vi "MicrowaveAmp.vi"(8 "error in (no error)":errorcluster, 11 "MicrowaveAmp in":refnum<class "MicrowaveAmp.lvclass">) -> (0 "error out":errorcluster, 3 "MicrowaveAmp out":refnum<class "MicrowaveAmp.lvclass">)   [LabVIEW 2009, in "MicrowaveAmp.lvclass"]
uses:
  MicrowaveAmp.lvclass
  Global/GPIB Numbers.vi
panel:
  out "Status":string
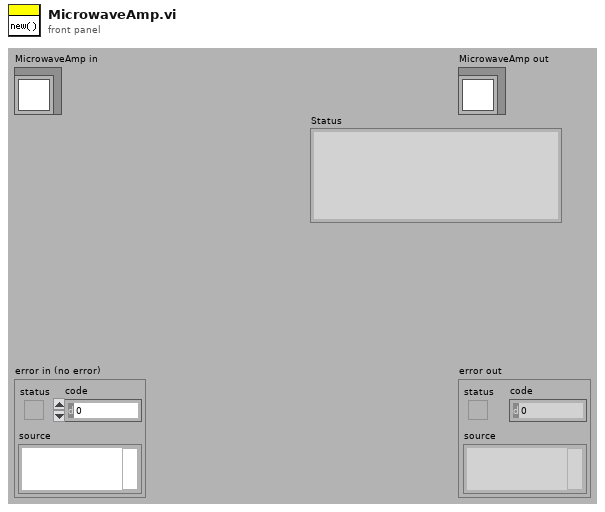
[diagram p1: front panel]
types:
  T1 = typedef "GPIB Type Def.ctl" = cluster{"Name":string, "bus":dbl, "GPIB":dbl, "GPIB as string":string, "byte":i32, "VISA Resource Name":refnum<visa-resource-name>}
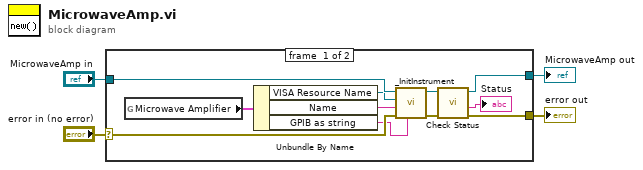
[diagram p0: block diagram]
diagram:
  n1 = case shown="No Error" "error in (no error)" {
    selector: "error in (no error)" -> [w13 w17]
    tunnel: [w11 w17] -> w3
    tunnel: [w9 w16] -> w1
    tunnel: "MicrowaveAmp in" -> [w14 w16]
    frame #0 {
      n2 = global read "GPIB Numbers.vi" "Microwave Amplifier"() -> (w15:T1)
      n3 = Unbundle By Name(w15) -> ("VISA Resource Name"=w7:refnum<visa-resource-name>, "Name"=w6:string, "GPIB as string"=w5:string)
      n4 = call-dynamic "_InitInstrument.vi"("GPIB as string"=w5, "error in (no error)"=w13, "Name"=w6, "VISA Resource Name"=w7, "Instrument in"=w14) -> ("error out"=w12:errorcluster, "Instrument out"=w10:refnum<class "MicrowaveAmp.lvclass">)  [unwired: 1 in, 4 out]
      n5 = call-dynamic "Check Status.vi"("error in (no error)"=w12, "MicrowaveAmp in"=w10) -> ("error out"=w11:errorcluster, "Status"=→"Status":string, "MicrowaveAmp out"=w9:refnum<class "MicrowaveAmp.lvclass">)  [unwired: 6 in, 1 out]
    }
    frame #1 {
    }
  }
  "error out" <- w3
  "MicrowaveAmp out" <- w1
